vi "Convert Calibration Point.vi"(8 "error in (no error)":errorcluster, 11 "DB Results":string[][](array[string])) -> (0 "error out":errorcluster, 3 "Conversion":T1[](array[typedef]))   [LabVIEW 2026, in "Analysis.lvlib"]
uses:
  Analysis/Analysis.lvlib
  controls/Messaging Payloads/Calibration Point Table Insert.ctl
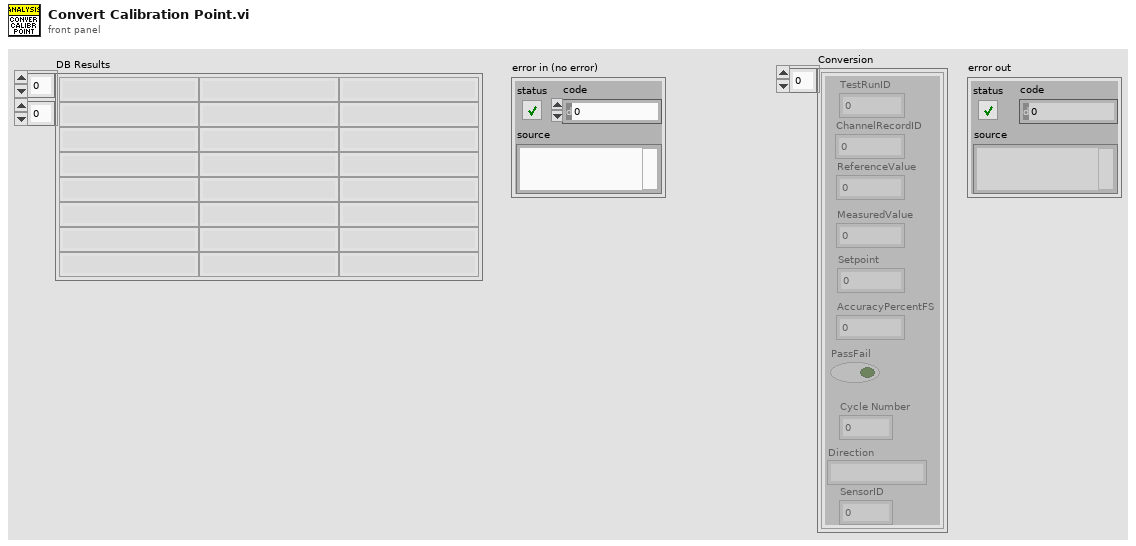
[diagram p1: front panel]
types:
  T1 = typedef "Calibration Point Table Insert.ctl" = cluster{"TestRunID":i32, "ChannelRecordID":i32, "Setpoint":dbl, "MeasuredValue":dbl, "AccuracyPercentFS":dbl, "PassFail":bool, "ReferenceValue":dbl, "Cycle Number":i32, "Direction":string, "SensorID":i32}
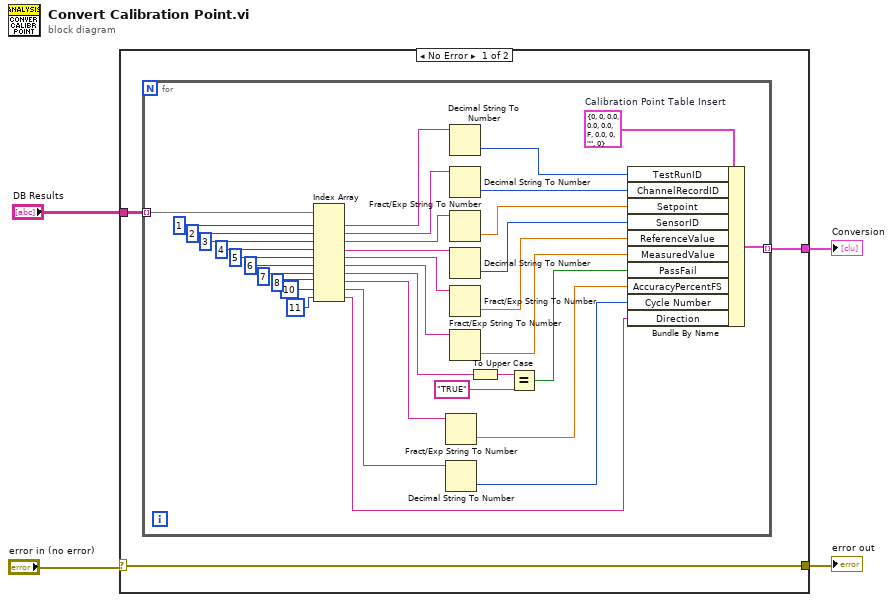
[diagram p0: block diagram]
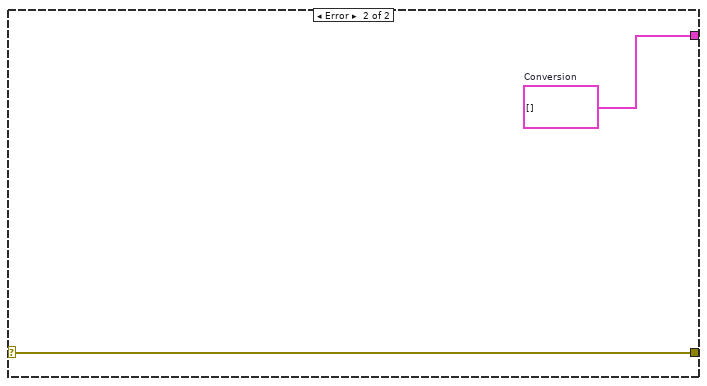
[diagram p2: hidden frame]
diagram:
  n1 = case shown="No Error" "error in (no error)" {
    selector: "error in (no error)" -> [w5 w43]
    tunnel: "DB Results" -> [w7 _]
    tunnel: [w6 w42] -> w3
    tunnel: [w5 w43] -> w1
    frame No Error {
      n2 = for {
        tunnel: w7 -> [w40] mode=indexing
        tunnel: [w9] -> w6 mode=indexing
        w41 = T1 {"TestRunID"=0, "ChannelRecordID"=0, "Setpoint"=0.0, "MeasuredValue"=0.0, "AccuracyPercentFS"=0.0, "PassFail"=FALSE, "ReferenceValue"=0.0, "Cycle Number"=0, "Direction"="", "SensorID"=0}  # Calibration Point Table Insert
        n3 = Index Array(array=w40, index #1=1 ("index"), index #2=2 ("index"), index #3=3 ("index"), index #4=4 ("index"), index #5=5 ("index"), index #6=6 ("index"), index #7=7 ("index"), index #8=8 ("index"), index #9=10 ("index"), index #10=11 ("index")) -> (element #1=w38:string, element #2=w35:string, element #3=w26:string, element #4=w29:string, element #5=w24:string, element #6=w21:string, element #7=w18:string, element #8=w14:string, element #9=w12:string, element #10=w10:string)
        n4 = Fract/Exp String To Number(string=w14) -> (number=w13:dbl)  [unwired: 3 in, 1 out]
        n5 = Decimal String To Number(string=w12) -> (number=w11:i32)  [unwired: 2 in, 1 out]
        n6 = Decimal String To Number(string=w38) -> (number=w37:i32)  [unwired: 2 in, 1 out]
        n7 = Decimal String To Number(string=w35) -> (number=w33:i32)  [unwired: 2 in, 1 out]
        n8 = Fract/Exp String To Number(string=w26) -> (number=w32:dbl)  [unwired: 3 in, 1 out]
        n9 = Decimal String To Number(string=w29) -> (number=w28:i32)  [unwired: 2 in, 1 out]
        n10 = Fract/Exp String To Number(string=w24) -> (number=w23:dbl)  [unwired: 3 in, 1 out]
        n11 = Fract/Exp String To Number(string=w21) -> (number=w20:dbl)  [unwired: 3 in, 1 out]
        n12 = To Upper Case(1:w18) -> (0:w17:string)
        n13 = Equal?(x=w17, y="TRUE") -> (x = y?=w15:bool)
        n14 = Bundle By Name(cluster=w41, "TestRunID"=w37, "ChannelRecordID"=w33, "Setpoint"=w32, "SensorID"=w28, "ReferenceValue"=w23, "MeasuredValue"=w20, "PassFail"=w15, "AccuracyPercentFS"=w13, "Cycle Number"=w11, "Direction"=w10) -> (w9:T1)
      }
    }
    frame Error {
      w42 = T1[] []  # Conversion
    }
  }
  "Conversion" <- w3
  "error out" <- w1
